vi "Set Discovery Info.vi"(8 "error in (no error)":errorcluster, 10 "Discovery Info":T1, 11 "Node in":refnum<class "Node Config.lvclass">) -> (0 "error out":errorcluster, 3 "Node out":refnum<class "Node Config.lvclass">)   [LabVIEW 2020, in "VectoConfig.lvlib" / "Node Config.lvclass"]
uses:
  Node Config.lvclass
  Discovery Info.ctl
  Node Config.lvclass/Node Config.ctl
  VectoConfig/VectoConfig.lvlib
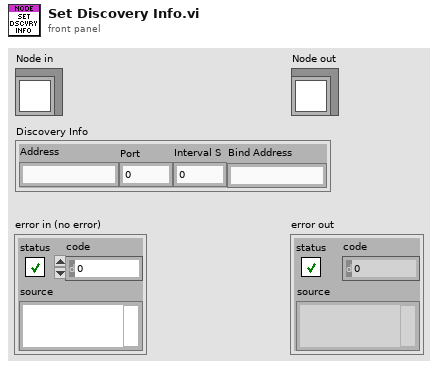
[diagram p1: front panel]
types:
  T1 = typedef "VectoConfig.lvlib/Discovery Info.ctl" = cluster{"Address":string, "Port":u16, "Interval S":dbl, "Bind Address":string}
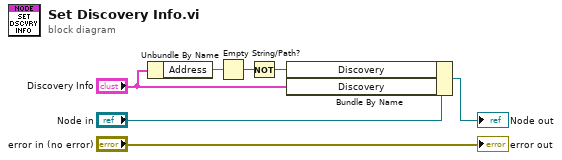
[diagram p0: block diagram]
diagram:
  n1 = Unbundle By Name("Discovery Info") -> ("Address"=w3:string)
  n2 = Empty String/Path?(string/path=w3) -> (empty?=w2:bool)
  n3 = Not(x=w2) -> (.not. x?=w1:bool)
  n4 = Bundle By Name(cluster="Node in", "Discovery"=w1, "Discovery"="Discovery Info") -> (→"Node out":refnum<class "Node Config.lvclass">)
  "error out" <- "error in (no error)"
